vi "Left Average Beacon Values (SubVI).vi"(8 "RB Y Center Array":dbl[](array[numeric]), 9 "RB X Center Array":dbl[](array[numeric]), 10 "LB Y Center Array":dbl[](array[numeric]), 11 "LB X Center Array":dbl[](array[numeric])) -> (0 "RB Y Center Array":dbl[](array[numeric]), 1 "RB X Center Array":dbl[](array[numeric]), 2 "LB Y Center Array":dbl[](array[numeric]), 3 "LB X Center Array":dbl[](array[numeric]))   [LabVIEW 2015]
uses:
  Left Variables.vi
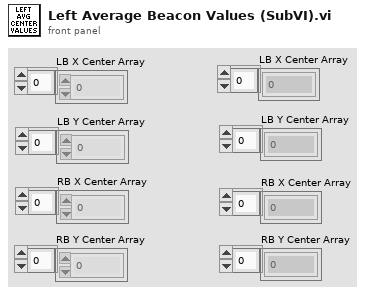
[diagram p1: front panel]
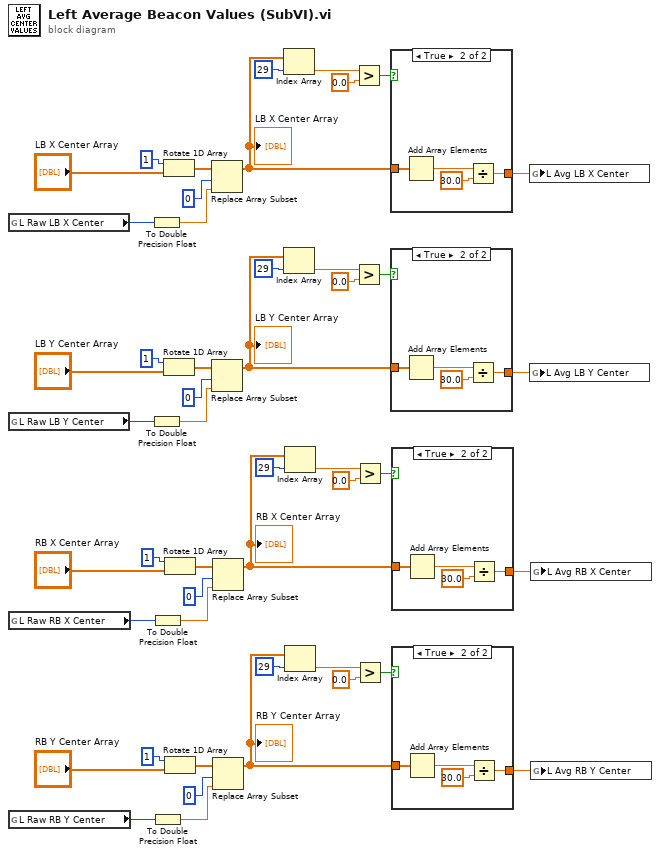
[diagram p0: block diagram]
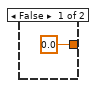
[diagram p2: hidden frame]
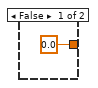
[diagram p3: hidden frame]
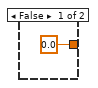
[diagram p4: hidden frame]
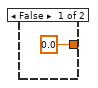
[diagram p5: hidden frame]
diagram:
  n1 = global read "Left Variables.vi" "L Raw LB X Center"() -> (w8:u16)
  n2 = global read "Left Variables.vi" "L Raw LB Y Center"() -> (w7:u16)
  n3 = global read "Left Variables.vi" "L Raw RB X Center"() -> (w6:u16)
  n4 = global read "Left Variables.vi" "L Raw RB Y Center"() -> (w5:u16)
  n5 = To Double Precision Float(number=w8) -> (double precision float=w10:dbl)
  n6 = To Double Precision Float(number=w7) -> (double precision float=w11:dbl)
  n7 = To Double Precision Float(number=w6) -> (double precision float=w12:dbl)
  n8 = To Double Precision Float(number=w5) -> (double precision float=w13:dbl)
  n9 = Rotate 1D Array(1:"LB X Center Array", 2:1 ("n")) -> (0:w19:dbl[])
  n10 = Rotate 1D Array(1:"LB Y Center Array", 2:1 ("n")) -> (0:w26:dbl[])
  n11 = Rotate 1D Array(1:"RB X Center Array", 2:1 ("n")) -> (0:w33:dbl[])
  n12 = Rotate 1D Array(1:"RB Y Center Array", 2:1 ("n")) -> (0:w40:dbl[])
  n13 = Replace Array Subset(array=w19, new element=w10, index=0) -> (w14:dbl[])
  "LB X Center Array" <- w14
  n14 = Replace Array Subset(array=w26, new element=w11, index=0) -> (w15:dbl[])
  "LB Y Center Array" <- w15
  n15 = Replace Array Subset(array=w33, new element=w12, index=0) -> (w16:dbl[])
  "RB X Center Array" <- w16
  n16 = Replace Array Subset(array=w40, new element=w13, index=0) -> (w17:dbl[])
  "RB Y Center Array" <- w17
  n17 = Index Array(array=w14, index=29) -> (element=w22:dbl)
  n18 = Index Array(array=w15, index=29) -> (element=w29:dbl)
  n19 = Index Array(array=w16, index=29) -> (element=w36:dbl)
  n20 = Index Array(array=w17, index=29) -> (element=w43:dbl)
  n21 = Greater?(x=w22, y=0.0) -> (0:w24:bool)
  n22 = Greater?(x=w29, y=0.0) -> (0:w31:bool)
  n23 = Greater?(x=w36, y=0.0) -> (0:w38:bool)
  n24 = Greater?(x=w43, y=0.0) -> (0:w45:bool)
  n25 = case shown="True" w24 {
    tunnel: [0.0 ("y") w50] -> w4
    tunnel: w14 -> [_ w53]
    frame False {
    }
    frame True {
      n26 = Add Array Elements(numeric array=w53) -> (sum=w52:dbl)
      n27 = Divide(x=w52, y=30.0) -> (x/y=w50:dbl)
    }
  }
  n28 = case shown="True" w31 {
    tunnel: [0.0 ("y") w55] -> w3
    tunnel: w15 -> [_ w58]
    frame False {
    }
    frame True {
      n29 = Add Array Elements(numeric array=w58) -> (sum=w57:dbl)
      n30 = Divide(x=w57, y=30.0) -> (x/y=w55:dbl)
    }
  }
  n31 = case shown="True" w38 {
    tunnel: [0.0 ("y") w60] -> w2
    tunnel: w16 -> [_ w63]
    frame False {
    }
    frame True {
      n32 = Add Array Elements(numeric array=w63) -> (sum=w62:dbl)
      n33 = Divide(x=w62, y=30.0) -> (x/y=w60:dbl)
    }
  }
  n34 = case shown="True" w45 {
    tunnel: [0.0 ("y") w65] -> w1
    tunnel: w17 -> [_ w68]
    frame False {
    }
    frame True {
      n35 = Add Array Elements(numeric array=w68) -> (sum=w67:dbl)
      n36 = Divide(x=w67, y=30.0) -> (x/y=w65:dbl)
    }
  }
  n37 = global write "Left Variables.vi" "L Avg LB X Center"(w4) -> ()
  n38 = global write "Left Variables.vi" "L Avg LB Y Center"(w3) -> ()
  n39 = global write "Left Variables.vi" "L Avg RB X Center"(w2) -> ()
  n40 = global write "Left Variables.vi" "L Avg RB Y Center"(w1) -> ()
